vi "SendMessageToLog2.vi"(7 "Log and view ?":T3, 8 "error in (no error)":errorcluster, 11 "Message":T1) -> (0 "error out":errorcluster)   [LabVIEW 2013]
uses:
  Ctrls/enumLogAndView.ctl
  030 - EVENTS/03 - ToMessageHandlerProcess/ToMessageHandlerEvent.ctl
  030 - EVENTS/03 - ToMessageHandlerProcess/enumMessageCriticity.ctl
  030 - EVENTS/EnumFgvEventCommand.ctl
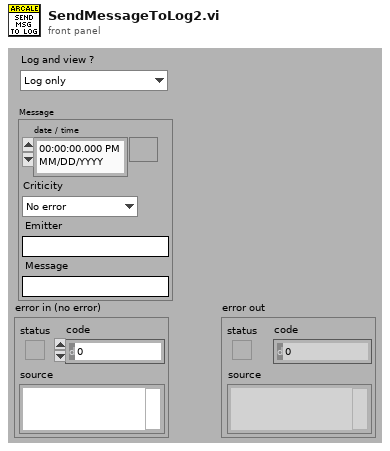
[diagram p1: front panel]
types:
  T1 = typedef "ToMessageHandlerEvent.ctl" = cluster{"date / time":timestamp, "Criticity":T2, "Emitter":string, "Message":string}
  T2 = typedef "enumMessageCriticity.ctl" = enum16{"No error", "Info", "Warning", "Error", "Fatal error"}
  T3 = typedef "enumLogAndView.ctl" = enum16{"Log only", "Log and view"}
  T4 = typedef "EnumFgvEventCommand.ctl" = enum16{"Setup", "Cleanup", "Get"}
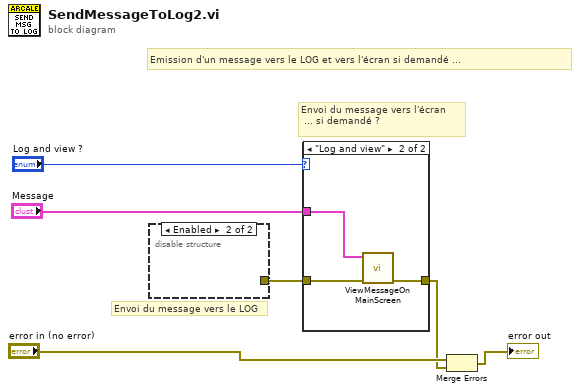
[diagram p0: block diagram]
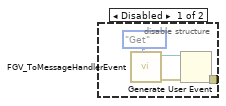
[diagram p2: hidden frame]
diagram:
  # "Envoi du message vers l'écran\n ... si demandé ?"
  # "Envoi du message vers le LOG"
  # "Emission d'un message vers le LOG et vers l'écran si demandé ..."
  n1 = disable-structure shown="Enabled" {
    disable-tunnel: [w7 _] -> w6
    frame Disabled {
      n2 = call "FGV_ToMessageHandlerEvent.vi"("Command"=EnumFgvEventCommand."Get") -> ("error out"=w9:errorcluster, "To message handler event"=w8:refnum<user-event>)  [unwired: 9 in]
      n3 = Generate User Event(user event=w8, error in=w9) -> (error out=w7:errorcluster)  [unwired: 2 in, 1 out]
    }
    frame Enabled {
    }
  }
  n4 = case shown="\"Log and view\"" "Log and view ?" {
    tunnel: w6 -> [w11 w14]
    tunnel: [w11 w13] -> w3
    tunnel: "Message" -> [_ w12]
    frame "Log only", Default {
    }
    frame "Log and view" {
      n5 = call "ViewMessageOnMainScreen.vi"("error in (no error)"=w14, "Message"=w12) -> ("error out"=w13:errorcluster)  [unwired: 9 in]
    }
  }
  n6 = Merge Errors("error in (no error)", w3) -> (→"error out":errorcluster)
